vi "create_plot.vi"(5 "Width per Box Plot":dbl=10.0 format="%.2f", 11 "Raw Box Plot Data":cluster{"Samples":dbl[]}[](array[cluster])) -> (2 "Number of Plots":i32, 3 "Box Plots":cluster{dbl[], dbl[]}[](array[cluster]))   [LabVIEW 2021, in "statistics.lvlib"]
uses:
  statistics.lvlib
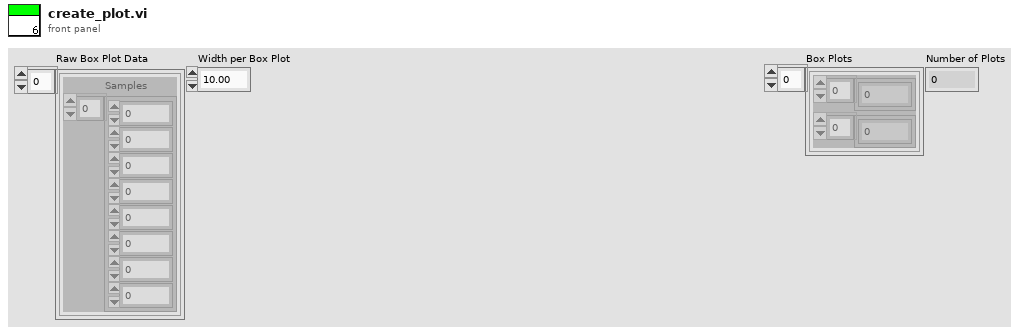
[diagram p1: front panel]
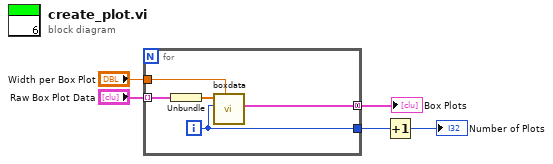
[diagram p0: block diagram]
diagram:
  n1 = for {
    tunnel: "Raw Box Plot Data" -> [w10] mode=indexing
    tunnel: [w9] -> w4 mode=concatenating
    tunnel: [w7] -> w3
    tunnel: "Width per Box Plot" -> [w6]
    i -> [w7]
    n2 = Unbundle(w10) -> ("Samples"=w8:dbl[])
    n3 = call "boxdata.vi"("Box Width"=w6, "Plot #"=w7, "Raw Data"=w8) -> ("XY Graph"=w9:cluster{dbl[], dbl[]}[])  [unwired: 8 in]
  }
  "Box Plots" <- w4
  n4 = Increment(x=w3) -> (x+1=→"Number of Plots":i32)
